vi "Close.vi"(8 "error in (no error)":errorcluster, 11 "pcap reference":u64) -> (0 "error out":errorcluster)   [LabVIEW 2025, in "Automotive Ethernet Bus Monitor UI.lvlib" / "lvwpcap.lvlib"]
doc: "This VI closes down the packet sniffing session denoted by pcap reference."
uses:
  lvwpcap.lvlib
  lvwpcap.dll
panel:
  # "Select Help»Show Context Help and move the cursor over the VI icon to display help for this VI."
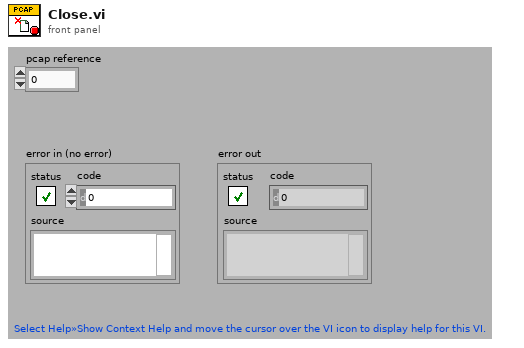
[diagram p1: front panel]
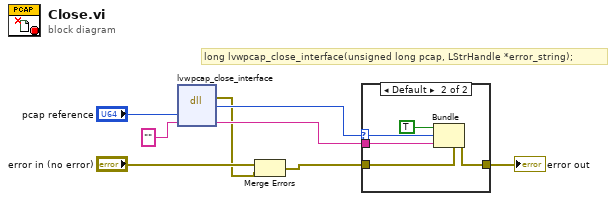
[diagram p0: block diagram]
diagram:
  # "long lvwpcap_close_interface(unsigned long pcap, LStrHandle *error_string);"
  n1 = dll-call lib="lvwpcap.*" fn="lvwpcap_close_interface"("pcap"="pcap reference", "error_string"="") -> (error out=w2:errorcluster, "return type"=w6:i32, "error_string"=w5:string)  [unwired: 4 in, 1 out]
  n2 = Merge Errors("error in (no error)", w2) -> (w3:errorcluster)
  n3 = case shown="Default" w6 {
    selector: w6 -> [_ w13]
    tunnel: w5 -> [_ w12]
    tunnel: w3 -> [w9 w14]
    tunnel: [w9 w10] -> w7
    frame 0 {
    }
    frame Default {
      n4 = Bundle(cluster=w14, "status"=TRUE, "code"=w13, "source"=w12) -> (w10:errorcluster)
    }
  }
  "error out" <- w7
